vi "Scale Timestamp.vi"(11 "Time Stamp":timestamp) -> (3 "Scaled timestamp":dbl)   [LabVIEW 2014, in "AcquisitionCoreObjects.lvlib" / "AcquistionObject.lvclass"]
uses:
  AcquistionObject.lvclass
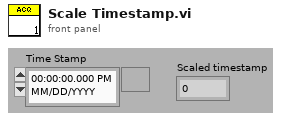
[diagram p1: front panel]
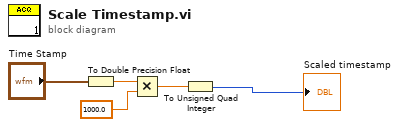
[diagram p0: block diagram]
diagram:
  n1 = To Double Precision Float(number="Time Stamp") -> (double precision float=w4:dbl)
  n2 = Multiply(x=w4, y=1000.0) -> (x*y=w3:dbl)
  n3 = To Unsigned Quad Integer(1:w3) -> (0:→"Scaled timestamp":u64)
